vi "Bundle AOL parameters.vi"(10 "AOL_Globals in":T1={"Imaging Protocol"=enum."AOL Z-Stack", "Number of POI"=0, "Number of Miniscans"=0, "Number of Trials"=0, "Number of Cycles "=0, "# Averaged Frames"=0, "Laser power (%)"=0, "Pockels (V)"=0.0, "Acquisition Length (sec)"=0.0, "Fill time (us)"=0.0, "POI Dwell time (us)"=0.0, "Miniscan Dwell time per pixel (us)"=0.0, "PMT 1"=0.0, "PMT 2"=0.0, "Back Apperture (mA)"=0.0, "Frame Size"=0, "Center Frequency"=0.0, "Field of View (um)"=175.0, "Field of View (norm)"=0.0, "DwellTime (us)"=0.0, "Ref Dwell Time (us)"=0.0, "Wavelength (nm)"=0.0, "Zoom"=0.0, "AOL Z"=0.0, "AOL Mode"=enum."Raster", "GridXY"=0.0, "GridZ"=0.0, "TriggerPeriod (sec)"=0.0, "Number of Pixels in Miniscan"=0, "Experiment folder path"=path "", "X centre"=0.0, "Y centre"=0.0, "Angle (degrees)"=0.0, "Angle Xs (degrees)"=0.0, "Angle Ys (degrees)"=0.0, "Plane Mode"=0, "Threshold"=[], "Regenerate Chirps"=FALSE, "Rectangle ROI length (pixels)"=0, "Rectangle ROI height (pixels)"=0, "AOD fill"=4900, "StartupDelay"=0, "Samples Wait after Trigger"=5080, "Slip Cycle"=600000, "Add Cycle"=TRUE, "Functional Mode"=enum."Point", "Z Start"=0.0, "Z Stop"=0.0, "# Planes"=0, "Total Pixels"=0, "Variable Miniscan Pixels"=[], "Use Variable Length"=FALSE, "Use Variable Resolution"=FALSE, "Laser power (%) at Z Start"=0, "Laser power (%) at Z Stop"=0, "Ref Z Step"=0} {"Angle Ys (degrees)" format="%#.6g"; "Angle Xs (degrees)" format="%#.6g"; "Plane Mode" items=["XY Plane", "XZ Plane", "YZ Plane", "arbitraryplane"]; "Frame Size" items=["100X100"=100, "128X128"=128, "200X200"=200, "256X256"=256, "512X512"=512, "1024x1024"=1024, "2048x2048"=2048]; "Back Apperture (mA)" format="%#.6g"; "Pockels (V)" format="%#.6g"; "PMT 2" format="%#.6g"; "PMT 1" format="%#.6g"; "Angle (degrees)" format="%#.6g"; "POI Dwell time (us)" format="%#.6g"}, 11 "Experiment folder path":path) -> (3 "AOL_Globals out":T1={"Imaging Protocol"=enum."AOL Z-Stack", "Number of POI"=0, "Number of Miniscans"=0, "Number of Trials"=0, "Number of Cycles "=0, "# Averaged Frames"=0, "Laser power (%)"=0, "Pockels (V)"=0.0, "Acquisition Length (sec)"=0.0, "Fill time (us)"=0.0, "POI Dwell time (us)"=0.0, "Miniscan Dwell time per pixel (us)"=0.0, "PMT 1"=0.0, "PMT 2"=0.0, "Back Apperture (mA)"=0.0, "Frame Size"=0, "Center Frequency"=0.0, "Field of View (um)"=175.0, "Field of View (norm)"=0.0, "DwellTime (us)"=0.0, "Ref Dwell Time (us)"=0.0, "Wavelength (nm)"=0.0, "Zoom"=0.0, "AOL Z"=0.0, "AOL Mode"=enum."Raster", "GridXY"=0.0, "GridZ"=0.0, "TriggerPeriod (sec)"=0.0, "Number of Pixels in Miniscan"=0, "Experiment folder path"=path "", "X centre"=0.0, "Y centre"=0.0, "Angle (degrees)"=0.0, "Angle Xs (degrees)"=0.0, "Angle Ys (degrees)"=0.0, "Plane Mode"=0, "Threshold"=[], "Regenerate Chirps"=FALSE, "Rectangle ROI length (pixels)"=0, "Rectangle ROI height (pixels)"=0, "AOD fill"=4900, "StartupDelay"=0, "Samples Wait after Trigger"=5080, "Slip Cycle"=600000, "Add Cycle"=TRUE, "Functional Mode"=enum."Point", "Z Start"=0.0, "Z Stop"=0.0, "# Planes"=0, "Total Pixels"=0, "Variable Miniscan Pixels"=[], "Use Variable Length"=FALSE, "Use Variable Resolution"=FALSE, "Laser power (%) at Z Start"=0, "Laser power (%) at Z Stop"=0, "Ref Z Step"=0} {"Angle Ys (degrees)" format="%#.6g"; "Angle Xs (degrees)" format="%#.6g"; "Plane Mode" items=["XY Plane", "XZ Plane", "YZ Plane", "arbitraryplane"]; "Frame Size" items=["100X100"=100, "128X128"=128, "200X200"=200, "256X256"=256, "512X512"=512, "1024x1024"=1024, "2048x2048"=2048]; "Back Apperture (mA)" format="%#.6g"; "Pockels (V)" format="%#.6g"; "PMT 2" format="%#.6g"; "PMT 1" format="%#.6g"; "Angle (degrees)" format="%#.6g"; "POI Dwell time (us)" format="%#.6g"})   [LabVIEW 2020]
uses:
  Typedefs/Controls/AOL_Globals.ctl
  Typedefs/Imaging Protocols enum.ctl
  Typedefs/Frame Size.ctl
  Typedefs/AOL modes.ctl
  Typedefs/Plane Mode.ctl
  Typedefs/Functional Mode.ctl
  Global Variables/General Globals.vi
  Global Variables/gl_UI Ctrl Refs.vi
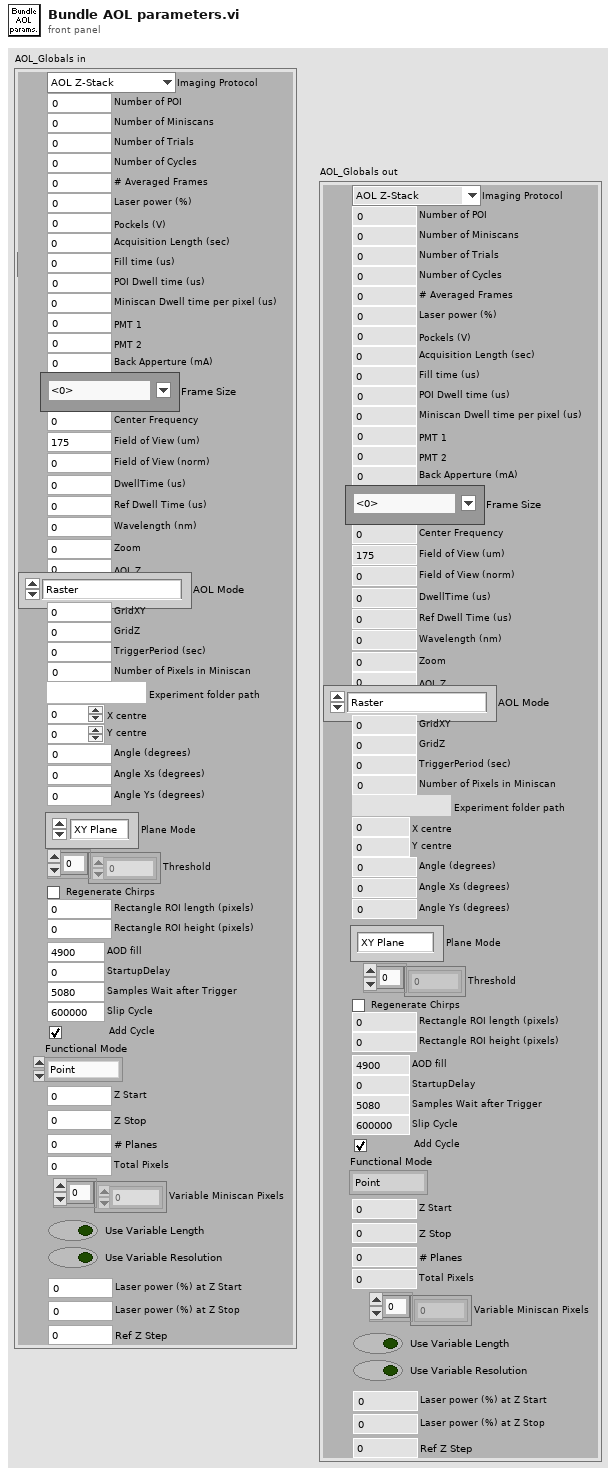
[diagram p1: front panel]
types:
  T1 = typedef "AOL_Globals.ctl" = cluster{"Imaging Protocol":T2, "Number of POI":u16, "Number of Miniscans":u16, "Number of Trials":u16, "Number of Cycles ":u64, "# Averaged Frames":u16, "Laser power (%)":u8, "Pockels (V)":dbl, "Acquisition Length (sec)":dbl, "Fill time (us)":dbl, "POI Dwell time (us)":dbl, "Miniscan Dwell time per pixel (us)":dbl, "PMT 1":dbl, "PMT 2":dbl, "Back Apperture (mA)":dbl, "Frame Size":T3, "Center Frequency":dbl, "Field of View (um)":dbl, "Field of View (norm)":dbl, "DwellTime (us)":dbl, "Ref Dwell Time (us)":dbl, "Wavelength (nm)":dbl, "Zoom":dbl, "AOL Z":dbl, "AOL Mode":T4, "GridXY":dbl, "GridZ":dbl, "TriggerPeriod (sec)":dbl, "Number of Pixels in Miniscan":u16, "Experiment folder path":path, "X centre":dbl, "Y centre":dbl, "Angle (degrees)":dbl, "Angle Xs (degrees)":dbl, "Angle Ys (degrees)":dbl, "Plane Mode":T5, "Threshold":u16[], "Regenerate Chirps":bool, "Rectangle ROI length (pixels)":u16, "Rectangle ROI height (pixels)":u16, "AOD fill":u16, "StartupDelay":i32, "Samples Wait after Trigger":u16, "Slip Cycle":u32, "Add Cycle":bool, "Functional Mode":T6, "Z Start":dbl, "Z Stop":dbl, "# Planes":i32, "Total Pixels":i32, "Variable Miniscan Pixels":u16[], "Use Variable Length":bool, "Use Variable Resolution":bool, "Laser power (%) at Z Start":u8, "Laser power (%) at Z Stop":u8, "Ref Z Step":i8}
  T2 = typedef "Imaging Protocols enum.ctl" = enum16{"AOL Z-Stack", "Motor Z Stack", "Parameter Sweep", "Functional Acquisition", "Single Plane Acquisition", "Volume Acquisition", "Live Imaging", "Live Plane Imaging", "Live Volume Imaging"}
  T3 = typedef "Frame Size.ctl" = u16
  T4 = typedef "AOL modes.ctl" = enum16{"Raster", "Structural", "Pointing", "Mini Scan", "Alignment"}
  T5 = typedef "Plane Mode.ctl" = u16
  T6 = typedef "Functional Mode.ctl" = enum16{"Point", "Line", "Patch", "Plane", "Volume"}
  T7 = typedef "UI ctrl refs cluster.ctl" = cluster{"Top level VI path":path, "Top level VI ref":refnum<vi>, "User menu ref":refnum<k9>, "Sub Panel control":refnum<vi>, "Imaging Param Tab":refnum<vi>, "Occurrence-Start drivers":refnum<k4>, "Occurrence-Speed logging initialised":refnum<k4>, "Occurrence-XYZ stage initialised":refnum<k4>, "Exit button":refnum<vi>, "Status ind":refnum<vi>, "Set as origin":refnum<vi>, "Speed Logging":refnum<vi>, "Time Lapse":refnum<vi>, "Live Imaging":refnum<vi>, "AOL Z Stack":refnum<vi>, "Motor Z Stack":refnum<vi>, "Funct Acq button":refnum<vi>, "Hard Shutter":refnum<vi>, "Virtual Shutter":refnum<vi>, "Laser Power":refnum<vi>, "AOL Mode":refnum<vi>, "Frame Size":refnum<vi>, "Field of View":refnum<vi>, "Dwell Time":refnum<vi>, "Zoom":refnum<vi>, "AOL Z":refnum<vi>, "Objective":refnum<vi>, "Axis":refnum<vi>, "Paths & Names":refnum<vi>, "Experiment folder path (ind.)":refnum<vi>, "Last State (Ind.)":refnum<vi>, "Averages":refnum<vi>, "Angle (degrees)":refnum<vi>, "X centre":refnum<vi>, "Y centre":refnum<vi>, "Plane Mode":refnum<vi>, "# Planes":refnum<vi>, "Z Start":refnum<vi>, "Z Stop":refnum<vi>, "Z Step":refnum<vi>, "PMT 1":refnum<vi>, "PMT 2":refnum<vi>, "Stage XYZ Position":refnum<vi>, "Pockels@Z Start":refnum<vi>, "Pockels@Z Stop":refnum<vi>, "Obtain Z Start":refnum<vi>, "Obtain Z Stop":refnum<vi>, "Live stim.trig.period":refnum<vi>, "Live stim.trig.enable":refnum<vi>, "Movement Correction":refnum<vi>, "Load Reference Image":refnum<vi>, "XY Stage Move":refnum<vi>, "MovCor Cluster":refnum<vi>, "RefDAQParam":refnum<vi>, "Funct. Acq. Pockels Modulation":refnum<vi>, "Ref Laser Power":refnum<vi>, "Enable Video Recording":refnum<vi>, "Video Record-Live Imaging":refnum<vi>, "Video Record-Funct acq":refnum<vi>, "Reference Source":refnum<vi>, "AOL Z-stack Chirps Ready (ind)":refnum<vi>, "Target time between mov.cor. ref triggers (ms)":refnum<vi>, "Funct. Acq. Ref frame save":refnum<vi>, "Tracking button":refnum<vi>, "Show ref plots window":refnum<vi>, "Center freq ind (nm)":refnum<vi>, "Pickup mode (ind)":refnum<vi>, "Logging queue (ind)":refnum<vi>, "Back aperture power (ind.)":refnum<vi>, "Power after objective (ind.)":refnum<vi>, "Switch user":refnum<vi>, "Ls1 Conn. Status":refnum<vi>, "Ls1Tuning Status":refnum<vi>, "Ls1 Faults":refnum<vi>, "Ls1 Connection":refnum<vi>, "Ls1 Mode":refnum<vi>, "Ls1 POWER [mW]":refnum<vi>, "Ls1Shutter":refnum<vi>, "Ls1 Wavelength":refnum<vi>, "Ls1 Note":refnum<vi>, "Ls1 Confirm Wav":refnum<vi>, "Ls1 PreChrp Prism1":refnum<vi>, "Ls1 PreChrp Prism2":refnum<vi>, "Ls1 wav top Ind":refnum<vi>, "Ls1 power top Ind":refnum<vi>, "Ls1 Pump peak Hold":refnum<vi>, "Ls1 Status Ind":refnum<vi>, "Ls1 wav cancel":refnum<vi>, "Experiment Type":refnum<vi>, "Biology Information":refnum<vi>, "Camera recording status":refnum<vi>, "Optimise Obj. Pos.":refnum<vi>}
  T8 = typedef "Laser control knob.ctl" = u16
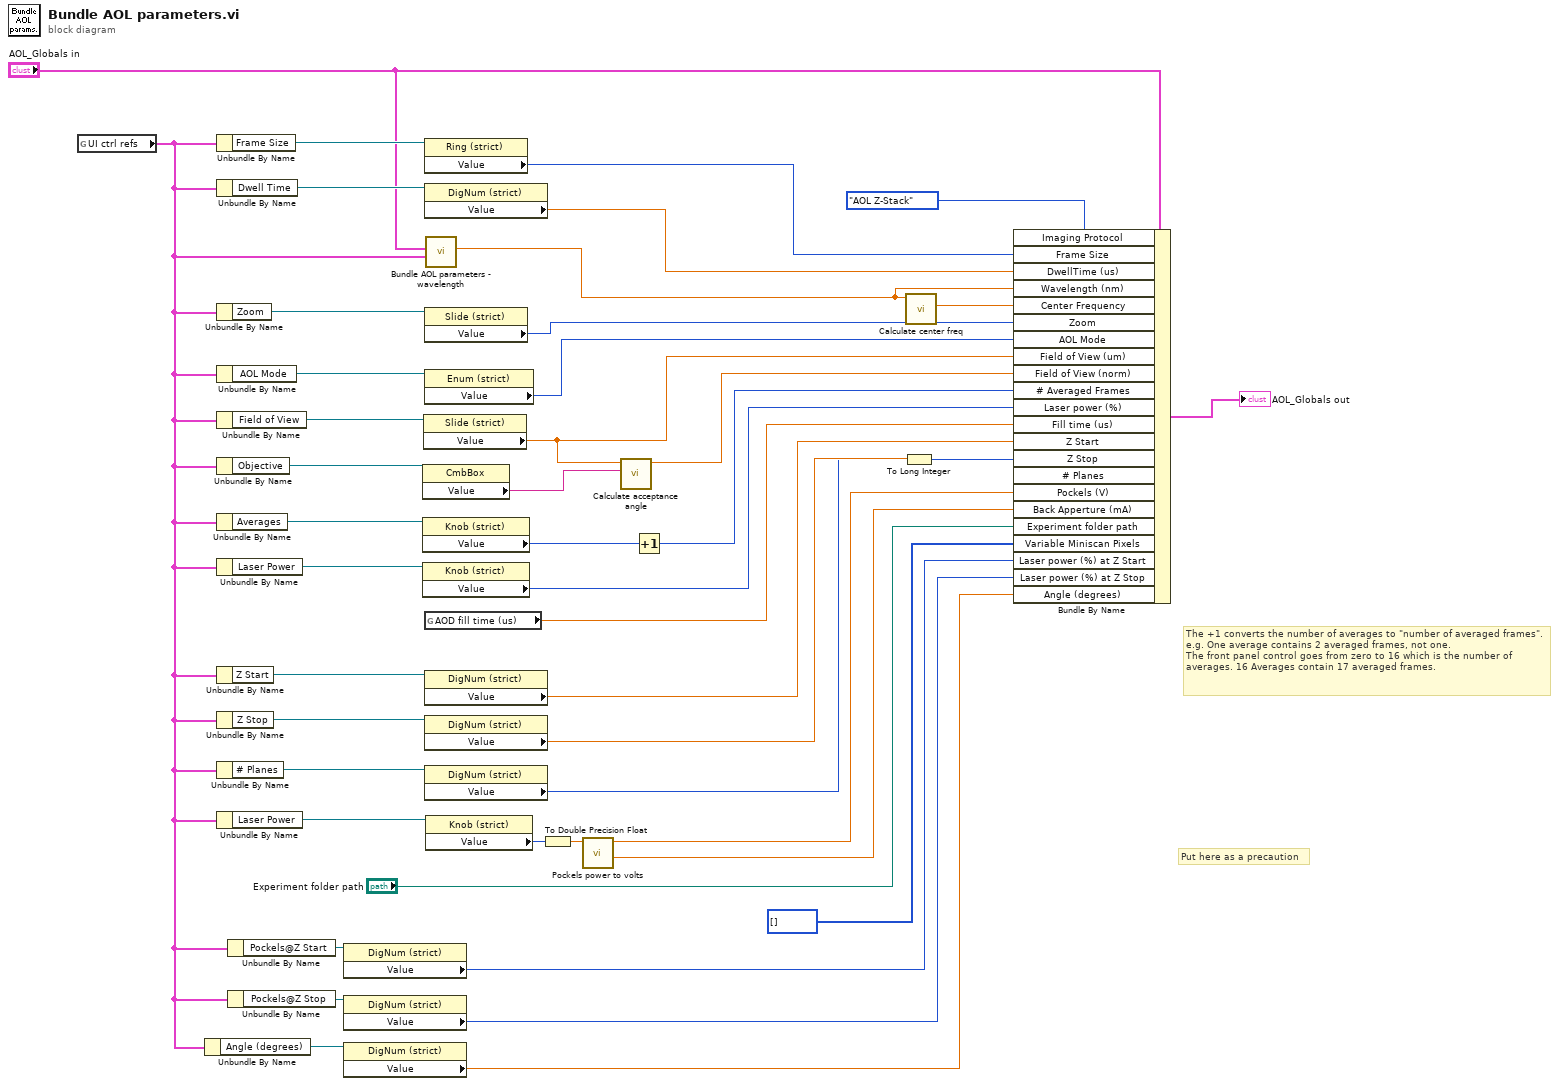
[diagram p0: block diagram]
diagram:
  # "Put here as a precaution"
  # "The +1 converts the number of averages to \"number of averaged frames\". e.g. One average contains 2 averaged frames, not one.\nThe front panel control goes from zero to 16 which is the number of averages. 16 Averages contain 17 averaged frames."
  n1 = global read "gl_UI Ctrl Refs.vi" "UI ctrl refs"() -> (w3:T7)
  n2 = Unbundle By Name(w3) -> ("Angle (degrees)"=w4:refnum<vi>)
  n3 = Unbundle By Name(w3) -> ("Frame Size"=w29:refnum<vi>)
  n4 = Unbundle By Name(w3) -> ("Dwell Time"=w31:refnum<vi>)
  n5 = Unbundle By Name(w3) -> ("Zoom"=w32:refnum<vi>)
  n6 = Unbundle By Name(w3) -> ("AOL Mode"=w27:refnum<vi>)
  n7 = Unbundle By Name(w3) -> ("Field of View"=w33:refnum<vi>)
  n8 = Unbundle By Name(w3) -> ("Objective"=w18:refnum<vi>)
  n9 = Unbundle By Name(w3) -> ("Averages"=w34:refnum<vi>)
  n10 = Unbundle By Name(w3) -> ("Laser Power"=w42:refnum<vi>)
  n11 = Unbundle By Name(w3) -> ("Z Start"=w39:refnum<vi>)
  n12 = Unbundle By Name(w3) -> ("Z Stop"=w38:refnum<vi>)
  n13 = Unbundle By Name(w3) -> ("# Planes"=w37:refnum<vi>)
  n14 = Unbundle By Name(w3) -> ("Laser Power"=w15:refnum<vi>)
  n15 = Unbundle By Name(w3) -> ("Pockels@Z Start"=w8:refnum<vi>)
  n16 = Unbundle By Name(w3) -> ("Pockels@Z Stop"=w7:refnum<vi>)
  n17 = property on="Property Node" class="DigNum (strict)"(reference=w8) -> ("Value"=w6:u16)  [unwired: 1 in, 2 out]
  n18 = property on="Property Node" class="DigNum (strict)"(reference=w7) -> ("Value"=w5:u16)  [unwired: 1 in, 2 out]
  n19 = property on="Property Node" class="DigNum (strict)"(reference=w4) -> ("Value"=w2:dbl)  [unwired: 1 in, 2 out]
  n20 = property on="Property Node" class="CmbBox"(reference=w18) -> ("Value"=w17:string)  [unwired: 1 in, 2 out]
  n21 = property class="Knob (strict)"(reference=w34) -> ("Value"=w36:u16)  [unwired: 1 in, 2 out]
  n22 = property class="Knob (strict)"(reference=w42) -> ("Value"=w43:T8)  [unwired: 1 in, 2 out]
  n23 = property class="Slide (strict)"(reference=w33) -> ("Value"=w1:sgl)  [unwired: 1 in, 2 out]
  n24 = property class="Ring (strict)"(reference=w29) -> ("Value"=w30:u16)  [unwired: 1 in, 2 out]
  n25 = property class="DigNum (strict)"(reference=w31) -> ("Value"=w35:dbl)  [unwired: 1 in, 2 out]
  n26 = property class="Slide (strict)"(reference=w32) -> ("Value"=w40:i8)  [unwired: 1 in, 2 out]
  n27 = property class="Enum (strict)"(reference=w27) -> ("Value"=w26:T4)  [unwired: 1 in, 2 out]
  n28 = global read "General Globals.vi" "AOD fill time (us)"() -> (w45:dbl)
  n29 = property class="DigNum (strict)"(reference=w39) -> ("Value"=w23:dbl)  [unwired: 1 in, 2 out]
  n30 = property class="DigNum (strict)"(reference=w38) -> ("Value"=w22:dbl)  [unwired: 1 in, 2 out]
  n31 = property class="DigNum (strict)"(reference=w37) -> ("Value"=w21:u16)  [unwired: 1 in, 2 out]
  n32 = call "Bundle AOL parameters - wavelength.vi"("UI ctrl refs"=w3, "AOL_Globals in"="AOL_Globals in") -> ("Wavelength"=w20:dbl)  [unwired: 9 in]
  n33 = property class="Knob (strict)"(reference=w15) -> ("Value"=w13:T8)  [unwired: 1 in, 2 out]
  n34 = To Double Precision Float(number=w13) -> (double precision float=w14:dbl)
  n35 = call "Pockels power to volts.vi"("Pockels power (%)"=w14) -> ("Back-aperture power (mW)"=w10:dbl, "Pockels control voltage (V)"=w11:dbl)  [unwired: 8 in, 1 out]
  n36 = call "Calculate acceptance angle.vi"("Objective"=w17, "FOV (true)"=w1) -> ("Acceptance Angle (mrad)"=w16:dbl)  [unwired: 8 in, 1 out]
  n37 = Increment(x=w36) -> (x+1=w44:u16)
  n38 = To Long Integer(number=w21) -> (32bit integer=w24:i32)
  n39 = call "Calculate center freq.vi"("UI Wavelength"=w20) -> ("Centre frequency (MHz)"=w25:dbl)  [unwired: 9 in, 1 out]
  n40 = Bundle By Name(cluster="AOL_Globals in", "Imaging Protocol"=Imaging_Protocols_enum."AOL Z-Stack" ("Imaging Mode"), "Frame Size"=w30, "DwellTime (us)"=w35, "Wavelength (nm)"=w20, "Center Frequency"=w25, "Zoom"=w40, "AOL Mode"=w26, "Field of View (um)"=w1, "Field of View (norm)"=w16, "# Averaged Frames"=w44, "Laser power (%)"=w43, "Fill time (us)"=w45, "Z Start"=w23, "Z Stop"=w22, "# Planes"=w24, "Pockels (V)"=w11, "Back Apperture (mA)"=w10, "Experiment folder path"="Experiment folder path", "Variable Miniscan Pixels"=u16[] [], "Laser power (%) at Z Start"=w6, "Laser power (%) at Z Stop"=w5, "Angle (degrees)"=w2) -> (→"AOL_Globals out":T1)
